vi "testpath2.vi"() -> (4 "Trajectory":T1[](array[typedef])=[{"t"=0.0, "velocity"=0.0, "acceleration"=2.3435826973687655, "pose"={"Translation2d"={"x"=0.0774192, "y"=0.185928}, "Rotation2d"={"Theta"=0.0}}, "curvature"=0.0}, {"t"=0.047106173277091413, "velocity"=0.11039721263144635, "acceleration"=-3.263996154199559, "pose"={"Translation2d"={"x"=0.08001852308776901, "y"=0.18586066416240327}, "Rotation2d"={"Theta"=-0.07810185233815048}}, "curvature"=-61.60474858569354}, {"t"=0.053259671361296806, "velocity"=0.0903122185497256, "acceleration"=-2.363925957623396, "pose"={"Translation2d"={"x"=0.08063303765779138, "y"=0.18579968634924657}, "Rotation2d"={"Theta"=-0.12154551781557862}}, "curvature"=-79.45370864068988}, {"t"=0.06060253182111065, "velocity"=0.07295424010556517, "acceleration"=-1.4416949338866047, "pose"={"Translation2d"={"x"=0.08122597127297766, "y"=0.1857117331972243}, "Rotation2d"={"Theta"=-0.1749375579100152}}, "curvature"=-99.06661763312775}, {"t"=0.0693110261969842, "velocity"=0.06039924788208828, "acceleration"=-0.9104988700910287, "pose"={"Translation2d"={"x"=0.08179438323477223, "y"=0.18559312894960375}, "Rotation2d"={"Theta"=-0.23853145947540738}}, "curvature"=-120.27826003101855}, {"t"=0.07938804352490185, "velocity"=0.05122413499113154, "acceleration"=-0.5792120596634627, "pose"={"Translation2d"={"x"=0.08233575624007373, "y"=0.18544072707720197}, "Rotation2d"={"Theta"=-0.31235747491337}}, "curvature"=-142.35551992491696}, {"t"=0.09077921007888227, "velocity"=0.04462623394943099, "acceleration"=-0.4038192359290258, "pose"={"Translation2d"={"x"=0.08284798009679452, "y"=0.18525188992348018}, "Rotation2d"={"Theta"=-0.3960059769552128}}, "curvature"=-163.8427702789242}, {"t"=0.09695072372373545, "velocity"=0.042134058024840826, "acceleration"=-0.31270644647916435, "pose"={"Translation2d"={"x"=0.08309260897132852, "y"=0.1851431179841045}, "Rotation2d"={"Theta"=-0.44121092624603003}}, "curvature"=-173.70999654118847}, {"t"=0.1033891694247334, "velocity"=0.0401207145488327, "acceleration"=-0.23490831082187247, "pose"={"Translation2d"={"x"=0.08332933543942006, "y"=0.18502446834963807}, "Rotation2d"={"Theta"=-0.488410728551556}}, "curvature"=-182.57657050349928}, {"t"=0.11005992609071186, "velocity"=0.03855369836852396, "acceleration"=-0.16695995975553915, "pose"={"Translation2d"={"x"=0.08355800297536588, "y"=0.18489574536915074}, "Rotation2d"={"Theta"=-0.5373459655625522}}, "curvature"=-190.11843445708558}, {"t"=0.116921657984853, "velocity"=0.037408063887624854, "acceleration"=-0.10600567598132761, "pose"={"Translation2d"={"x"=0.08377847744456844, "y"=0.18475678137970777}, "Rotation2d"={"Theta"=-0.5877071696426507}}, "curvature"=-196.03207220702802}, {"t"=0.12392714615426638, "velocity"=0.036665442378646995, "acceleration"=-0.0496073097812525, "pose"={"Translation2d"={"x"=0.0839906465946472, "y"=0.18460743607027907}, "Rotation2d"={"Theta"=-0.6391410543429555}}, "curvature"=-200.06281680826004}, {"t"=0.1310246385654173, "velocity"=0.03631335487393694, "acceleration"=0.004395319498262556, "pose"={"Translation2d"={"x"=0.08419441954654981, "y"=0.18444759584564838}, "Rotation2d"={"Theta"=-0.6912605824921103}}, "curvature"=-202.03146098771143}, {"t"=0.13815963801809006, "velocity"=0.03634471547615137, "acceleration"=0.05799027336927698, "pose"={"Translation2d"={"x"=0.08438972628566341, "y"=0.18427717319032236}, "Rotation2d"={"Theta"=-0.7436582689510874}}, "curvature"=-201.85456553695633}, {"t"=0.14527697526679556, "velocity"=0.03675745180886514, "acceleration"=0.11307728618805102, "pose"={"Translation2d"={"x"=0.0845765171529258, "y"=0.18409610603243998}, "Rotation2d"={"Theta"=-0.7959215893197124}}, "curvature"=-199.55457553174037}, {"t"=0.1523229647059073, "velocity"=0.037554193173149564, "acceleration"=0.17153717059604345, "pose"={"Translation2d"={"x"=0.08475476233593672, "y"=0.18390435710768158}, "Rotation2d"={"Theta"=-0.8476489989740198}}, "curvature"=-195.25769330622686}, {"t"=0.15924742526920344, "velocity"=0.038741995546081265, "acceleration"=0.23529206064245542, "pose"={"Translation2d"={"x"=0.08492445136006903, "y"=0.18370191332317803}, "Rotation2d"={"Theta"=-0.8984649589344123}}, "curvature"=-189.17993139104587}, {"t"=0.1660053740784075, "velocity"=0.04033208724711512, "acceleration"=0.3063602871556492, "pose"={"Translation2d"={"x"=0.08508559257958, "y"=0.1834887851214201}, "Rotation2d"={"Theta"=-0.9480325468739267}}, "curvature"=-181.6041156418403}, {"t"=0.17255825778502296, "velocity"=0.042339630581171406, "acceleration"=0.386908937568493, "pose"={"Translation2d"={"x"=0.0852382126687225, "y"=0.1832650058441675}, "Rotation2d"={"Theta"=-0.9960626519615907}}, "curvature"=-172.8521201807349}, {"t"=0.1788746609843625, "velocity"=0.0447835034322821, "acceleration"=0.47930689894890155, "pose"={"Translation2d"={"x"=0.08538235611285627, "y"=0.1830306310963581}, "Rotation2d"={"Theta"=-1.042319298697744}}, "curvature"=-163.2569342559984}, {"t"=0.18493050448955045, "velocity"=0.04768611100327358, "acceleration"=0.6490919973330421, "pose"={"Translation2d"={"x"=0.0855180846995591, "y"=0.18278573811001714}, "Rotation2d"={"Theta"=-1.0866211858450743}}, "curvature"=-153.1383845294613}, {"t"=0.19615830692266117, "velocity"=0.0549739877102422, "acceleration"=0.941459206443059, "pose"={"Translation2d"={"x"=0.08576462790874101, "y"=0.18226481066873368}, "Rotation2d"={"Theta"=-1.168895958568751}}, "curvature"=-132.44212851381863}, {"t"=0.20622279984151345, "velocity"=0.06444929722687665, "acceleration"=1.3418311536022953, "pose"={"Translation2d"={"x"=0.0859786633034792, "y"=0.18170324974681615}, "Rotation2d"={"Theta"=-1.2424085833564584}}, "curvature"=-112.53274117550998}, {"t"=0.21513918561432827, "velocity"=0.07641358143437582, "acceleration"=1.8923758205411287, "pose"={"Translation2d"={"x"=0.08616125615759282, "y"=0.18110238689435}, "Rotation2d"={"Theta"=-1.3072572259381148}}, "curvature"=-94.44693395075514}, {"t"=0.22297099217614624, "velocity"=0.09123430280311551, "acceleration"=2.6528140193058642, "pose"={"Translation2d"={"x"=0.08631369972706873, "y"=0.18046383863010146}, "Rotation2d"={"Theta"=-1.363907802949199}}, "curvature"=-78.62059191289242}, {"t"=0.22980662803577084, "velocity"=0.10936797344239757, "acceleration"=3.652890312976089, "pose"={"Translation2d"={"x"=0.0864374989656209, "y"=0.1797894860866117}, "Rotation2d"={"Theta"=-1.4130182829288853}}, "curvature"=-65.0912298694915}, {"t"=0.23575071787636012, "velocity"=0.1310810816405457, "acceleration"=4.389436457462054, "pose"={"Translation2d"={"x"=0.08653435424024987, "y"=0.17908145465529096}, "Rotation2d"={"Theta"=-1.4553132146872143}}, "curvature"=-53.67673857261736}, {"t"=0.24564788073800228, "velocity"=0.17452404913087727, "acceleration"=4.999999999999998, "pose"={"Translation2d"={"x"=0.08665491372552997, "y"=0.17757395585970945}, "Rotation2d"={"Theta"=-1.5222489468742197}}, "curvature"=-36.06210546716506}, {"t"=0.2611381435219113, "velocity"=0.25197536305042223, "acceleration"=5.000000000000002, "pose"={"Translation2d"={"x"=0.0866654015927572, "y"=0.17427067852316036}, "Rotation2d"={"Theta"=-1.601097292473268}}, "curvature"=-14.158339729780822}, {"t"=0.27358680122956974, "velocity"=0.3142186515887145, "acceleration"=-4.755099044000396, "pose"={"Translation2d"={"x"=0.0865021887608069, "y"=0.17075028219178084}, "Rotation2d"={"Theta"=-1.6249193382438698}}, "curvature"=-2.6727087142999493e-14}, {"t"=0.28596110166702643, "velocity"=0.2553776274083906, "acceleration"=-5.000000000000002, "pose"={"Translation2d"={"x"=0.0863389759288566, "y"=0.16722988586040133}, "Rotation2d"={"Theta"=-1.6010972924732687}}, "curvature"=14.158339729780678}, {"t"=0.3011563859447309, "velocity"=0.17940120601986828, "acceleration"=-4.932206251410714, "pose"={"Translation2d"={"x"=0.08634946379608383, "y"=0.1639266085238522}, "Rotation2d"={"Theta"=-1.5222489468742206}}, "curvature"=36.062105467164734}, {"t"=0.31088799373988385, "velocity"=0.13140290921633757, "acceleration"=-3.711994416551717, "pose"={"Translation2d"={"x"=0.08647002328136393, "y"=0.16241910972827067}, "Rotation2d"={"Theta"=-1.4553132146872154}}, "curvature"=53.676738572616834}, {"t"=0.31682413838376733, "velocity"=0.10936797344239868, "acceleration"=-2.652814019305907, "pose"={"Translation2d"={"x"=0.08656687855599289, "y"=0.16171107829694997}, "Rotation2d"={"Theta"=-1.4130182829288873}}, "curvature"=65.09122986949086}, {"t"=0.3236597742433918, "velocity"=0.09123430280311662, "acceleration"=-1.8923758205411012, "pose"={"Translation2d"={"x"=0.08669067779454505, "y"=0.1610367257534602}, "Rotation2d"={"Theta"=-1.3639078029492022}}, "curvature"=78.62059191289143}, {"t"=0.33149158080521013, "velocity"=0.07641358143437649, "acceleration"=-1.3418311536023326, "pose"={"Translation2d"={"x"=0.08684312136402099, "y"=0.16039817748921165}, "Rotation2d"={"Theta"=-1.307257225938117}}, "curvature"=94.44693395075427}, {"t"=0.34040796657802436, "velocity"=0.06444929722687776, "acceleration"=-0.9414592064431023, "pose"={"Translation2d"={"x"=0.0870257142181346, "y"=0.1597973146367455}, "Rotation2d"={"Theta"=-1.2424085833564629}}, "curvature"=112.53274117550862}, {"t"=0.3504724594968764, "velocity"=0.05497398771024309, "acceleration"=-0.6490919973330328, "pose"={"Translation2d"={"x"=0.08723974961287277, "y"=0.15923575371482798}, "Rotation2d"={"Theta"=-1.1688959585687553}}, "curvature"=132.44212851381695}, {"t"=0.3617002619299876, "velocity"=0.047686111003274245, "acceleration"=-0.4793068989489879, "pose"={"Translation2d"={"x"=0.0874862928220547, "y"=0.1587148262735445}, "Rotation2d"={"Theta"=-1.0866211858450798}}, "curvature"=153.13838452945902}, {"t"=0.3677561054351754, "velocity"=0.04478350343228232, "acceleration"=-0.38690893756843653, "pose"={"Translation2d"={"x"=0.08762202140875751, "y"=0.15846993328720355}, "Rotation2d"={"Theta"=-1.0423192986977496}}, "curvature"=163.2569342559969}, {"t"=0.37407250863451474, "velocity"=0.04233963058117207, "acceleration"=-0.30636028715561286, "pose"={"Translation2d"={"x"=0.08776616485289127, "y"=0.15823555853939414}, "Rotation2d"={"Theta"=-0.9960626519616004}}, "curvature"=172.8521201807327}, {"t"=0.38062539234113096, "velocity"=0.04033208724711579, "acceleration"=-0.23529206064256067, "pose"={"Translation2d"={"x"=0.0879187849420338, "y"=0.1580117792621415}, "Rotation2d"={"Theta"=-0.9480325468739346}}, "curvature"=181.60411564183696}, {"t"=0.3873833411503339, "velocity"=0.03874199554608149, "acceleration"=-0.1715371705960183, "pose"={"Translation2d"={"x"=0.08807992616154474, "y"=0.1577986510603836}, "Rotation2d"={"Theta"=-0.8984649589344227}}, "curvature"=189.17993139104385}, {"t"=0.3943078017136297, "velocity"=0.03755419317315001, "acceleration"=-0.11307728618807471, "pose"={"Translation2d"={"x"=0.08824961518567706, "y"=0.15759620727588008}, "Rotation2d"={"Theta"=-0.8476489989740267}}, "curvature"=195.25769330622353}, {"t"=0.40135379115274195, "velocity"=0.03675745180886536, "acceleration"=-0.05799027336924636, "pose"={"Translation2d"={"x"=0.08842786036868798, "y"=0.15740445835112166}, "Rotation2d"={"Theta"=-0.795921589319721}}, "curvature"=199.55457553173815}, {"t"=0.4084711284014474, "velocity"=0.03634471547615181, "acceleration"=-0.004395319498231251, "pose"={"Translation2d"={"x"=0.08861465123595037, "y"=0.15722339119323928}, "Rotation2d"={"Theta"=-0.7436582689510949}}, "curvature"=201.8545655369545}, {"t"=0.41560612785412043, "velocity"=0.03631335487393761, "acceleration"=0.04960730978122319, "pose"={"Translation2d"={"x"=0.088809957975064, "y"=0.15705296853791326}, "Rotation2d"={"Theta"=-0.6912605824921199}}, "curvature"=202.03146098770893}, {"t"=0.4227036202652711, "velocity"=0.03666544237864744, "acceleration"=0.10600567598136021, "pose"={"Translation2d"={"x"=0.08901373092696659, "y"=0.15689312831328253}, "Rotation2d"={"Theta"=-0.6391410543429665}}, "curvature"=200.06281680825916}, {"t"=0.4297091084346844, "velocity"=0.03740806388762552, "acceleration"=0.16695995975550962, "pose"={"Translation2d"={"x"=0.08922590007704534, "y"=0.15674378300385383}, "Rotation2d"={"Theta"=-0.587707169642665}}, "curvature"=196.0320722070255}, {"t"=0.4365708403288254, "velocity"=0.0385536983685244, "acceleration"=0.23490831082185235, "pose"={"Translation2d"={"x"=0.0894463745462479, "y"=0.15660481901441087}, "Rotation2d"={"Theta"=-0.5373459655625644}}, "curvature"=190.1184344570844}, {"t"=0.44324159699480353, "velocity"=0.040120714548832925, "acceleration"=0.31270644647914475, "pose"={"Translation2d"={"x"=0.0896750420821937, "y"=0.15647609603392354}, "Rotation2d"={"Theta"=-0.48841072855157025}}, "curvature"=182.57657050349698}, {"t"=0.4496800426958012, "velocity"=0.042134058024840826, "acceleration"=0.4038192359289669, "pose"={"Translation2d"={"x"=0.08991176855028524, "y"=0.15635744639945712}, "Rotation2d"={"Theta"=-0.4412109262460405}}, "curvature"=173.70999654118788}, {"t"=0.4558515563406553, "velocity"=0.04462623394943099, "acceleration"=0.5792120596635256, "pose"={"Translation2d"={"x"=0.09015639742481926, "y"=0.1562486744600814}, "Rotation2d"={"Theta"=-0.39600597695523054}}, "curvature"=163.8427702789235}, {"t"=0.4672427228946352, "velocity"=0.05122413499113199, "acceleration"=0.9104988700909966, "pose"={"Translation2d"={"x"=0.09066862128154003, "y"=0.15605983730635964}, "Rotation2d"={"Theta"=-0.31235747491338145}}, "curvature"=142.35551992491614}, {"t"=0.47731974022255297, "velocity"=0.0603992478820885, "acceleration"=1.4416949338865988, "pose"={"Translation2d"={"x"=0.09120999428684154, "y"=0.15590743543395782}, "Rotation2d"={"Theta"=-0.23853145947542465}}, "curvature"=120.27826003101823}, {"t"=0.4860282345984264, "velocity"=0.07295424010556517, "acceleration"=2.3639259576235054, "pose"={"Translation2d"={"x"=0.09177840624863609, "y"=0.15578883118633724}, "Rotation2d"={"Theta"=-0.17493755791003093}}, "curvature"=99.06661763312779}, {"t"=0.4933710950582401, "velocity"=0.09031221854972604, "acceleration"=3.0164280995608284, "pose"={"Translation2d"={"x"=0.09237133986382236, "y"=0.15570087803431498}, "Rotation2d"={"Theta"=-0.1215455178155994}}, "curvature"=79.45370864068965}, {"t"=0.4995676187072388, "velocity"=0.10900358660415899, "acceleration"=3.2099466552372213, "pose"={"Translation2d"={"x"=0.09298585443384472, "y"=0.15563990022115828}, "Rotation2d"={"Theta"=-0.07810185233816763}}, "curvature"=61.60474858569303}, {"t"=0.5182710790606299, "velocity"=0.16904069660688842, "acceleration"=-3.716363985732206, "pose"={"Translation2d"={"x"=0.09558517752161375, "y"=0.1555725643835615}, "Rotation2d"={"Theta"=-1.8307092179778333e-14}}, "curvature"=-1.7250053967029693e-12}, {"t"=0.5377224922029448, "velocity"=0.09675216533319107, "acceleration"=-2.770464533483307, "pose"={"Translation2d"={"x"=0.09816917506467329, "y"=0.1556453832888355}, "Rotation2d"={"Theta"=0.08595677451778284}}, "curvature"=70.17784975737536}, {"t"=0.5446559894788898, "velocity"=0.07754315703718229, "acceleration"=-2.0078311841616534, "pose"={"Translation2d"={"x"=0.09876980402437249, "y"=0.1557113264441974}, "Rotation2d"={"Theta"=0.1350468581629947}}, "curvature"=93.02774184231959}, {"t"=0.5530595181598164, "velocity"=0.060670290094621215, "acceleration"=-1.1912172586961445, "pose"={"Translation2d"={"x"=0.09934270232277766, "y"=0.15580644150438278}, "Rotation2d"={"Theta"=0.19658385081852184}}, "curvature"=119.72761813837175}, {"t"=0.5632492336568042, "velocity"=0.04853212513340566, "acceleration"=-0.8124403499649132, "pose"={"Translation2d"={"x"=0.09988408692354683, "y"=0.15593470353810518}, "Rotation2d"={"Theta"=0.2715148453026896}}, "curvature"=150.41695984182707}, {"t"=0.5690825133830074, "velocity"=0.04379293331120593, "acceleration"=-0.6349231723740711, "pose"={"Translation2d"={"x"=0.10014192836966991, "y"=0.15601234978286024}, "Rotation2d"={"Theta"=0.3142341701670356}}, "curvature"=167.0170658151397}, {"t"=0.5753905930993192, "velocity"=0.03978778732613675, "acceleration"=-0.4948018649167662, "pose"={"Translation2d"={"x"=0.10039071755097403, "y"=0.15609951529223298}, "Rotation2d"={"Theta"=0.36050711576775285}}, "curvature"=184.12921053172292}, {"t"=0.5821688812682085, "velocity"=0.03643387769922701, "acceleration"=-0.38270215664740254, "pose"={"Translation2d"={"x"=0.10063013081876065, "y"=0.15619653959569954}, "Rotation2d"={"Theta"=0.4102979234949966}}, "curvature"=201.35329274080783}, {"t"=0.5894020159674006, "velocity"=0.03366574145052503, "acceleration"=-0.29170994164656977, "pose"={"Translation2d"={"x"=0.10085987584071117, "y"=0.156303729204168}, "Rotation2d"={"Theta"=0.46349009309414674}}, "curvature"=218.15424122373147}, {"t"=0.5970616394795439, "velocity"=0.03143135312276302, "acceleration"=-0.2165495287954919, "pose"={"Translation2d"={"x"=0.101079690949347, "y"=0.1564213582978653}, "Rotation2d"={"Theta"=0.5198699448216428}}, "curvature"=233.87405185452747}, {"t"=0.6051047522811616, "velocity"=0.029689620835523733, "acceleration"=-0.1530548516883707, "pose"={"Translation2d"={"x"=0.10128934449048972, "y"=0.15654966941422405}, "Rotation2d"={"Theta"=0.5791145438826865}}, "curvature"=247.7688931629093}, {"t"=0.6134730769029672, "velocity"=0.028408808151653142, "acceleration"=-0.09781653921956363, "pose"={"Translation2d"={"x"=0.101488634171721, "y"=0.15668887413576937}, "Rotation2d"={"Theta"=0.6407871610915417}}, "curvature"=259.0738230220722}, {"t"=0.6220938211947187, "velocity"=0.027565556779537204, "acceleration"=-0.047936377452372066, "pose"={"Translation2d"={"x"=0.10167738641084273, "y"=0.15683915377800575}, "Rotation2d"={"Theta"=0.7043431189362696}}, "curvature"=267.090182633088}, {"t"=0.630882063228603, "velocity"=0.027144280292258127, "acceleration"=-0.0008482709654389815, "pose"={"Translation2d"={"x"=0.10185545568433707, "y"=0.1570006600773038}, "Rotation2d"={"Theta"=0.7691476236098189}}, "curvature"=271.2816109003646}, {"t"=0.6397446945257157, "velocity"=0.027136762379451396, "acceleration"=0.04581900522136835, "pose"={"Translation2d"={"x"=0.1020227238758265, "y"=0.1571735158787871}, "Rotation2d"={"Theta"=0.8345050811793381}}, "curvature"=271.35759117150434}, {"t"=0.6485855194035324, "velocity"=0.02754184018068928, "acceleration"=0.094352224676927, "pose"={"Translation2d"={"x"=0.10217909962453388, "y"=0.1573578158242192}, "Rotation2d"={"Theta"=0.8996969187800623}}, "curvature"=267.3227413392821}, {"t"=0.6573108246167323, "velocity"=0.028365092138539882, "acceleration"=0.1470463333023926, "pose"={"Translation2d"={"x"=0.10232451767374248, "y"=0.15755362703989023}, "Rotation2d"={"Theta"=0.9640228667260538}}, "curvature"=259.4776945641172}, {"t"=0.665834611580665, "velocity"=0.02961848375743692, "acceleration"=0.20628477568028816, "pose"={"Translation2d"={"x"=0.10245893821925611, "y"=0.15776098982450382}, "Rotation2d"={"Theta"=1.0268397706121175}}, "curvature"=248.3711315953599}, {"t"=0.6740827724095978, "velocity"=0.03131995376380825, "acceleration"=0.27461105367069044, "pose"={"Translation2d"={"x"=0.10258234625785909, "y"=0.15797991833706393}, "Rotation2d"={"Theta"=1.0875926461201102}}, "curvature"=234.7164907677842}, {"t"=0.6819957548250865, "velocity"=0.033492946202603235, "acceleration"=0.35479413019379735, "pose"={"Translation2d"={"x"=0.10269475093577635, "y"=0.15821040128476174}, "Rotation2d"={"Theta"=1.1458346067318121}}, "curvature"=219.2950955053735}, {"t"=0.6895295990710837, "velocity"=0.03616590991887736, "acceleration"=0.44989007893007565, "pose"={"Translation2d"={"x"=0.1027961848971335, "y"=0.1584524026108624}, "Rotation2d"={"Theta"=1.201234763455286}}, "curvature"=202.86726425582916}, {"t"=0.6966555302806612, "velocity"=0.03937179567320448, "acceleration"=0.5633026373286869, "pose"={"Translation2d"={"x"=0.10288670363241685, "y"=0.15870586218259194}, "Rotation2d"={"Theta"=1.2535754049780008}}, "curvature"=186.10613248202148}, {"t"=0.7033584784246697, "velocity"=0.04314758404060193, "acceleration"=0.69884590081536, "pose"={"Translation2d"={"x"=0.1029663848269335, "y"=0.15897069647902398}, "Rotation2d"={"Theta"=1.3027411728436478}}, "curvature"=169.55964344713635}, {"t"=0.7096349582300072, "velocity"=0.047533876224112426, "acceleration"=0.8608132364314004, "pose"={"Translation2d"={"x"=0.1030353277092714, "y"=0.1592467992789667}, "Rotation2d"={"Theta"=1.3487034150678574}}, "curvature"=153.63837147221966}, {"t"=0.7154907009894446, "velocity"=0.05257457710057345, "acceleration"=1.1710273135760545, "pose"={"Translation2d"={"x"=0.10309365239975934, "y"=0.15953404234884963}, "Rotation2d"={"Theta"=1.3915026250306544}}, "curvature"=138.62245564664414}, {"t"=0.7259394069127965, "velocity"=0.06481029712834241, "acceleration"=1.7215619926356163, "pose"={"Translation2d"={"x"=0.10317902823596548, "y"=0.16014133042958176}, "Rotation2d"={"Theta"=1.4680178073712176}}, "curvature"=111.88933562608142}, {"t"=0.7349184761898326, "velocity"=0.08026832152493002, "acceleration"=2.491621101203314, "pose"={"Translation2d"={"x"=0.10322386637448248, "y"=0.1607911207447828}, "Rotation2d"={"Theta"=1.5333858309580801}}, "curvature"=89.768286926723}, {"t"=0.7426047973908486, "velocity"=0.0994197216200079, "acceleration"=3.320618702108264, "pose"={"Translation2d"={"x"=0.10322981342353883, "y"=0.16148166514471396}, "Rotation2d"={"Theta"=1.5889293086419294}}, "curvature"=71.90243531656316}, {"t"=0.755075794176805, "velocity"=0.14083114678138683, "acceleration"=5.00000000000001, "pose"={"Translation2d"={"x"=0.10313295843700387, "y"=0.1629766148075767}, "Rotation2d"={"Theta"=1.675700032982173}}, "curvature"=46.28096736583443}, {"t"=0.7650105898872683, "velocity"=0.19050512533370356, "acceleration"=4.999999999999997, "pose"={"Translation2d"={"x"=0.1029066952555758, "y"=0.16460686722462275}, "Rotation2d"={"Theta"=1.7372462719476571}}, "curvature"=29.907284772497857}, {"t"=0.78087148876621, "velocity"=0.2698096197284119, "acceleration"=5.0, "pose"={"Translation2d"={"x"=0.1021549388228159, "y"=0.16817912604026272}, "Rotation2d"={"Theta"=1.808119721975475}}, "curvature"=11.392762400320894}, {"t"=0.7938746162185758, "velocity"=0.3348252569902407, "acceleration"=-4.87580343734334, "pose"={"Translation2d"={"x"=0.10117532587401734, "y"=0.17198618356164386}, "Rotation2d"={"Theta"=1.8300183745307927}}, "curvature"=0.33963534680191004}, {"t"=0.8224893227987234, "velocity"=0.1953055722881857, "acceleration"=-5.000000000000001, "pose"={"Translation2d"={"x"=0.0994219257031623, "y"=0.17936549989866496}, "Rotation2d"={"Theta"=1.7435098835081544}}, "curvature"=-28.695429879989835}, {"t"=0.8321101400212955, "velocity"=0.1472014861753257, "acceleration"=-3.737334957184971, "pose"={"Translation2d"={"x"=0.09918347402379073, "y"=0.18099575231571102}, "Rotation2d"={"Theta"=1.6841931776688102}}, "curvature"=-44.681687822810645}, {"t"=0.8441274989785668, "velocity"=0.10228859045127559, "acceleration"=-2.6661130356198317, "pose"={"Translation2d"={"x"=0.09907192127589325, "y"=0.18249070197857378}, "Rotation2d"={"Theta"=1.6001259710533695}}, "curvature"=-69.80228261669235}, {"t"=0.851607676765601, "velocity"=0.08234559094450966, "acceleration"=-1.838290850505451, "pose"={"Translation2d"={"x"=0.09906961498842175, "y"=0.1831812463785049}, "Rotation2d"={"Theta"=1.5461204056689324}}, "curvature"=-87.42865136904975}, {"t"=0.8603672639780126, "velocity"=0.06624292191772896, "acceleration"=-1.2483239554812005, "pose"={"Translation2d"={"x"=0.09910561901369269, "y"=0.18383103669370598}, "Rotation2d"={"Theta"=1.4823867426308317}}, "curvature"=-109.4051223052071}, {"t"=0.8705912402278141, "velocity"=0.053480087444830904, "acceleration"=-0.8318978310404131, "pose"={"Translation2d"={"x"=0.09918159830382774, "y"=0.1844383247744381}, "Rotation2d"={"Theta"=1.4075396162448133}}, "curvature"=-136.224917991435}, {"t"=0.8824436182677277, "velocity"=0.04362011986075576, "acceleration"=-0.5998518589850211, "pose"={"Translation2d"={"x"=0.09929892660045758, "y"=0.1850016706442638}, "Rotation2d"={"Theta"=1.32036282084814}}, "curvature"=-167.69054870808148}, {"t"=0.8890509169113168, "velocity"=0.0396567194865296, "acceleration"=-0.47956032045977043, "pose"={"Translation2d"={"x"=0.09937344116172195, "y"=0.18526650494069583}, "Rotation2d"={"Theta"=1.2719031149668187}}, "curvature"=-184.74761053814296}, {"t"=0.8960938025586663, "velocity"=0.036279230988525146, "acceleration"=-0.37909202474885084, "pose"={"Translation2d"={"x"=0.09945866558544372, "y"=0.18551996451242536}, "Rotation2d"={"Theta"=1.2201732587521341}}, "curvature"=-202.22429069675667}, {"t"=0.9035615184878253, "velocity"=0.03344827943669104, "acceleration"=-0.29482779660640884, "pose"={"Translation2d"={"x"=0.09955468040193201, "y"=0.185761965838526}, "Rotation2d"={"Theta"=1.165256443743712}}, "curvature"=-219.59191832860543}, {"t"=0.9114297200747205, "velocity"=0.03112851489957169, "acceleration"=-0.22353499147615324, "pose"={"Translation2d"={"x"=0.09966154403160041, "y"=0.18599244878622384}, "Rotation2d"={"Theta"=1.107337414513009}}, "curvature"=-236.1782993686969}, {"t"=0.9196586026064402, "velocity"=0.02928907171298545, "acceleration"=-0.16230327944072007, "pose"={"Translation2d"={"x"=0.09977929213342746, "y"=0.18621137729878398}, "Rotation2d"={"Theta"=1.0467162157481573}}, "curvature"=-251.19803495847782}, {"t"=0.9281920121728392, "velocity"=0.027904071355548066, "acceleration"=-0.10848051716776347, "pose"={"Translation2d"={"x"=0.09990793695341624, "y"=0.18641874008339754}, "Rotation2d"={"Theta"=0.9838145805699998}}, "curvature"=-263.81388801484485}, {"t"=0.936957981706207, "velocity"=0.026953134447091465, "acceleration"=-0.05960573119375002, "pose"={"Translation2d"={"x"=0.10004746667305481, "y"=0.18661455129906857}, "Rotation2d"={"Theta"=0.9191717247022588}}, "curvature"=-273.22659999761464}, {"t"=0.9458709774559114, "velocity"=0.02642186881830355, "acceleration"=-0.01333662403488536, "pose"={"Translation2d"={"x"=0.10019784475777607, "y"=0.18679885124450066}, "Rotation2d"={"Theta"=0.8534274890519126}}, "curvature"=-278.7802541019173}, {"t"=0.9548358472267702, "velocity"=0.0263023077206479, "acceleration"=0.032631042753267656, "pose"={"Translation2d"={"x"=0.10035900930541793, "y"=0.186971707045984}, "Rotation2d"={"Theta"=0.7872929428384702}}, "curvature"=-280.06102787176684}, {"t"=0.9637530921406602, "velocity"=0.026593286720674403, "acceleration"=0.08065556213396426, "pose"={"Translation2d"={"x"=0.10053087239468307, "y"=0.18713321334528205}, "Rotation2d"={"Theta"=0.7215112626164386}}, "curvature"=-276.9640671721246}, {"t"=0.9725247548891591, "velocity"=0.027300770110504136, "acceleration"=0.13325800247006186, "pose"={"Translation2d"={"x"=0.10071331943359957, "y"=0.18728349298751842}, "Rotation2d"={"Theta"=0.6568140938882268}}, "curvature"=-269.7095376623658}, {"t"=0.9810600533034425, "velocity"=0.028438166927677422, "acceleration"=0.19325589530700452, "pose"={"Translation2d"={"x"=0.10090620850798024, "y"=0.18742269770906375}, "Rotation2d"={"Theta"=0.5938797909916752}}, "curvature"=-258.8032881521894}, {"t"=0.98927995564165, "velocity"=0.030026711513383875, "acceleration"=0.26393579962518937, "pose"={"Translation2d"={"x"=0.10110936972988338, "y"=0.18755100882542255}, "Rotation2d"={"Theta"=0.5332994383480658}}, "curvature"=-244.95392013920517}, {"t"=0.9971201652520616, "velocity"=0.03209602350613694, "acceleration"=0.3492878526136228, "pose"={"Translation2d"={"x"=0.1013226045860724, "y"=0.18766863791911984}, "Rotation2d"={"Theta"=0.4755545834395076}}, "curvature"=-228.9691317443559}, {"t"=1.0045323503304004, "velocity"=0.03468500971532462, "acceleration"=0.4543407293916066, "pose"={"Translation2d"={"x"=0.10154568528647583, "y"=0.18777582752758828}, "Rotation2d"={"Theta"=0.42100792629471184}}, "curvature"=-211.65596129145138}, {"t"=1.0114837920876667, "velocity"=0.03784333283364427, "acceleration"=0.5856615279390037, "pose"={"Translation2d"={"x"=0.10177835411264778, "y"=0.18787285183105482}, "Rotation2d"={"Theta"=0.36990573115040026}}, "curvature"=-193.74308696394925}, {"t"=1.017955843288908, "velocity"=0.04163376422906273, "acceleration"=0.7521310839980412, "pose"={"Translation2d"={"x"=0.10202032276622766, "y"=0.18796001734042758}, "Rotation2d"={"Theta"=0.32238910169977497}}, "curvature"=-175.8331728878996}, {"t"=1.0239416646425101, "velocity"=0.04613588653236622, "acceleration"=1.1077846736780808, "pose"={"Translation2d"={"x"=0.10227127171740036, "y"=0.18803766358518265}, "Rotation2d"={"Theta"=0.27851067991036266}}, "curvature"=-158.3840879145007}, {"t"=1.0343945509271988, "velocity"=0.05771543375424404, "acceleration"=1.875703575631341, "pose"={"Translation2d"={"x"=0.10279867232675113, "y"=0.18816592561890508}, "Rotation2d"={"Theta"=0.2015502334025794}}, "curvature"=-126.00976743551827}, {"t"=1.0430080981166385, "velocity"=0.0738718950163455, "acceleration"=2.467321293545936, "pose"={"Translation2d"={"x"=0.1033573503145702, "y"=0.18826104067909044}, "Rotation2d"={"Theta"=0.13838031277314014}}, "curvature"=-97.79899632033535}, {"t"=1.0501433849548638, "velocity"=0.09147694016785679, "acceleration"=3.253927227246253, "pose"={"Translation2d"={"x"=0.1039435586528987, "y"=0.18832698383445234}, "Rotation2d"={"Theta"=0.08802956458905108}}, "curvature"=-73.67639668026254}, {"t"=1.061422853396756, "velocity"=0.12817950963979463, "acceleration"=4.289933588494223, "pose"={"Translation2d"={"x"=0.10518074616443314, "y"=0.1883902483890585}, "Rotation2d"={"Theta"=0.02220021162876268}}, "curvature"=-34.51484544057754}, {"t"=1.0701857218783168, "velocity"=0.16577163347039933, "acceleration"=-3.6515252670326634, "pose"={"Translation2d"={"x"=0.10646863832853012, "y"=0.18839980273972629}, "Rotation2d"={"Theta"=2.9426732770626766e-14}}, "curvature"=2.836228175771673e-12}, {"t"=1.0895659679151655, "velocity"=0.09500417538553715, "acceleration"=-2.7207734633231833, "pose"={"Translation2d"={"x"=0.10899459853675333, "y"=0.1883290945273587}, "Rotation2d"={"Theta"=-0.0854011037217413}}, "curvature"=-71.36631849517777}, {"t"=1.096462169489461, "velocity"=0.07624117314446655, "acceleration"=-1.9934423590169708, "pose"={"Translation2d"={"x"=0.10958158763091988, "y"=0.1882650627678044}, "Rotation2d"={"Theta"=-0.13420095994761355}}, "curvature"=-94.66724584083127}, {"t"=1.1048161257058737, "velocity"=0.05958804295729614, "acceleration"=-1.182546116555915, "pose"={"Translation2d"={"x"=0.11014137547317829, "y"=0.18817270466588526}, "Rotation2d"={"Theta"=-0.19540776415030497}}, "curvature"=-121.95621322978805}, {"t"=1.1149542882556525, "velocity"=0.04759919820504277, "acceleration"=-0.8065776143012836, "pose"={"Translation2d"={"x"=0.11067024973438806, "y"=0.18804816037227076}, "Rotation2d"={"Theta"=-0.26999442698449216}}, "curvature"=-153.42344179030619}, {"t"=1.120762814474175, "velocity"=0.04291417098510042, "acceleration"=-0.6304787092517313, "pose"={"Translation2d"={"x"=0.11092208018326222, "y"=0.1879727647433057}, "Rotation2d"={"Theta"=-0.31254883046411347}}, "curvature"=-170.49808634267168}, {"t"=1.1270480150924895, "velocity"=0.03895148581187735, "acceleration"=-0.49156069935597885, "pose"={"Translation2d"={"x"=0.11116503003703918, "y"=0.1878881257704365}, "Rotation2d"={"Theta"=-0.3586707903789192}}, "curvature"=-188.1464616868444}, {"t"=1.1338064055172965, "velocity"=0.03562932668813845, "acceleration"=-0.38052086652499706, "pose"={"Translation2d"={"x"=0.11139878151500279, "y"=0.18779391376562116}, "Rotation2d"={"Theta"=-0.4083328422356733}}, "curvature"=-205.96732356101813}, {"t"=1.1410238482082429, "velocity"=0.03288293914128504, "acceleration"=-0.2905024408316854, "pose"={"Translation2d"={"x"=0.11162304753029403, "y"=0.1876898311023257}, "Rotation2d"={"Theta"=-0.46142764864700314}}, "curvature"=-223.4184511929345}, {"t"=1.1486732571737868, "velocity"=0.030660767165874736, "acceleration"=-0.21627825514852766, "pose"={"Translation2d"={"x"=0.11183757105163113, "y"=0.18757561154757615}, "Rotation2d"={"Theta"=-0.5177510355035749}}, "curvature"=-239.82676442283454}, {"t"=1.1567128479476634, "velocity"=0.02892197850119249, "acceleration"=-0.15372576433392146, "pose"={"Translation2d"={"x"=0.11204212446502954, "y"=0.1874510195940104}, "Rotation2d"={"Theta"=-0.5769891409471083}}, "curvature"=-254.42417091056544}, {"t"=1.1650853706883255, "velocity"=0.027634906043481067, "acceleration"=-0.09947696645275515, "pose"={"Translation2d"={"x"=0.11223650893552208, "y"=0.18731584979193017}, "Rotation2d"={"Theta"=-0.6387129060337343}}, "curvature"=-266.41245216187883}, {"t"=1.173718733856308, "velocity"=0.02677608526524522, "acceleration"=-0.05067511975014293, "pose"={"Translation2d"={"x"=0.11242055376887898, "y"=0.1871699260813528}, "Rotation2d"={"Theta"=-0.7023828897284227}}, "curvature"=-275.05292254920397}, {"t"=1.18252826789836, "velocity"=0.026329661072721278, "acceleration"=-0.004797565338293713, "pose"={"Translation2d"={"x"=0.11259411577332792, "y"=0.1870131011240634}, "Rotation2d"={"Theta"=-0.7673662089061012}}, "curvature"=-279.7669845299291}, {"t"=1.191420595654658, "velocity"=0.026286999549300916, "acceleration"=0.04047994497850446, "pose"={"Translation2d"={"x"=0.11275707862127413, "y"=0.18684525563566656}, "Rotation2d"={"Theta"=-0.8329653207785566}}, "curvature"=-280.22585487406246}, {"t"=1.2002987300489298, "velocity"=0.02664638594109281, "acceleration"=0.08739231833729783, "pose"={"Translation2d"={"x"=0.11290935221102039, "y"=0.1866662977176383}, "Rotation2d"={"Theta"=-0.8984558337431857}}, "curvature"=-276.4062167927869}, {"t"=1.2090677192116492, "velocity"=0.027412728233497496, "acceleration"=0.13817658257504883, "pose"={"Translation2d"={"x"=0.11305087202848717, "y"=0.18647616218937801}, "Rotation2d"={"Theta"=-0.9631283452570846}}, "curvature"=-268.59583728225317}, {"t"=1.2176400167928687, "velocity"=0.02859721901808676, "acceleration"=0.19515119988682209, "pose"={"Translation2d"={"x"=0.11318159850893261, "y"=0.1862748099202605}, "Rotation2d"={"Theta"=-1.0263282697065548}}, "curvature"=-257.34731321790406}, {"t"=1.2259398283000917, "velocity"=0.030216937192555804, "acceleration"=0.2607867143590383, "pose"={"Translation2d"={"x"=0.11330151639867268, "y"=0.18606222716168763}, "Rotation2d"={"Theta"=-1.0874881475790634}}, "curvature"=-243.39310723257265}, {"t"=1.2339059430997878, "velocity"=0.032294394097375445, "acceleration"=0.33777028458058916, "pose"={"Translation2d"={"x"=0.11341063411680115, "y"=0.18583842487914046}, "Rotation2d"={"Theta"=-1.1461488074139536}}, "curvature"=-227.54438118828813}, {"t"=1.2414929062649822, "velocity"=0.034857044804785575, "acceleration"=0.4290664247446799, "pose"={"Translation2d"={"x"=0.11350898311690968, "y"=0.18560343808423113}, "Rotation2d"={"Theta"=-1.2019682666495493}}, "curvature"=-210.5966476375705}, {"t"=1.248670698187739, "velocity"=0.037936794322644074, "acceleration"=0.5379765174373194, "pose"={"Translation2d"={"x"=0.11359661724880796, "y"=0.18535732516675463}, "Rotation2d"={"Theta"=-1.2547195637493243}}, "curvature"=-193.2584432255869}, {"t"=1.2554232926419575, "velocity"=0.04156953157079113, "acceleration"=0.6682002217051316, "pose"={"Translation2d"={"x"=0.11367361212024363, "y"=0.1851001672267409}, "Rotation2d"={"Theta"=-1.3042802230553217}}, "curvature"=-176.10946914655926}, {"t"=1.2617465343181247, "velocity"=0.0457947230607012, "acceleration"=0.8239027139112283, "pose"={"Translation2d"={"x"=0.11374006445862243, "y"=0.18483206740650665}, "Rotation2d"={"Theta"=-1.3506165973360953}}, "curvature"=-159.58620878017567}, {"t"=1.2676457409083308, "velocity"=0.05065509538029511, "acceleration"=1.122391568580036, "pose"={"Translation2d"={"x"=0.1137960914727283, "y"=0.1845531502227073}, "Rotation2d"={"Theta"=-1.3937660908844118}}, "curvature"=-143.9881381698022}, {"t"=1.2781700699034757, "velocity"=0.06246751350940816, "acceleration"=1.6527080595663284, "pose"={"Translation2d"={"x"=0.11387743694046792, "y"=0.18396346469503988}, "Rotation2d"={"Theta"=-1.4709054934935915}}, "curvature"=-116.19731747125384}, {"t"=1.2872111565072826, "velocity"=0.07740979020675676, "acceleration"=2.395385233282257, "pose"={"Translation2d"={"x"=0.11391897156665912, "y"=0.1833325088817287}, "Rotation2d"={"Theta"=-1.5367982374777287}}, "curvature"=-93.19314674514915}, {"t"=1.29494734435199, "velocity"=0.09594094033186695, "acceleration"=3.204427407084343, "pose"={"Translation2d"={"x"=0.11392230524663283, "y"=0.1826619802615057}, "Rotation2d"={"Theta"=-1.5927777102801357}}, "curvature"=-74.61756469850788}, {"t"=1.3015976260182398, "velocity"=0.1172512851680278, "acceleration"=3.9635813891197857, "pose"={"Translation2d"={"x"=0.11388931430289642, "y"=0.18195385417950594}, "Rotation2d"={"Theta"=-1.640176953540165}}, "curvature"=-59.793915573356564}, {"t"=1.3073961780550554, "velocity"=0.14023431810499237, "acceleration"=4.888068532447168, "pose"={"Translation2d"={"x"=0.1138221210601756, "y"=0.18121036247292885}, "Rotation2d"={"Theta"=-1.6802112971716348}}, "curvature"=-47.99961164993872}, {"t"=1.3171441949421774, "velocity"=0.1878832927046974, "acceleration"=5.000000000000002, "pose"={"Translation2d"={"x"=0.11359472443802737, "y"=0.1796273637491305}, "Rotation2d"={"Theta"=-1.742227843591752}}, "curvature"=-31.015296379228783}, {"t"=1.332779334450521, "velocity"=0.26605899024641594, "acceleration"=4.999999999999998, "pose"={"Translation2d"={"x"=0.11284541269991404, "y"=0.17615864866727718}, "Rotation2d"={"Theta"=-1.8137452147475845}}, "curvature"=-11.860679682631737}, {"t"=1.3456030394623133, "velocity"=0.3301775153053772, "acceleration"=-4.910842396854063, "pose"={"Translation2d"={"x"=0.11187097444868144, "y"=0.17246194063926945}, "Rotation2d"={"Theta"=-1.8361458971072673}}, "curvature"=-0.4762604750853638}, {"t"=1.3738990866630907, "velocity"=0.19122008704841614, "acceleration"=-5.0, "pose"={"Translation2d"={"x"=0.11011795218492636, "y"=0.16529651752940838}, "Rotation2d"={"Theta"=-1.7507804064940407}}, "curvature"=29.308064752294065}, {"t"=1.383473390431305, "velocity"=0.14334856820734476, "acceleration"=-3.6369410802705238, "pose"={"Translation2d"={"x"=0.10987436072510647, "y"=0.16371351880561003}, "Rotation2d"={"Theta"=-1.691817044899504}}, "curvature"=45.74029558457744}, {"t"=1.3954555702468752, "velocity"=0.09977008620490979, "acceleration"=-2.6282295167646774, "pose"={"Translation2d"={"x"=0.10975464764669657, "y"=0.16226190101703314}, "Rotation2d"={"Theta"=-1.6080938154691242}}, "curvature"=71.63947680773273}, {"t"=1.4029083334522467, "velocity"=0.0801825139670942, "acceleration"=-1.8082331049564886, "pose"={"Translation2d"={"x"=0.10974701513166105, "y"=0.16159137239681015}, "Rotation2d"={"Theta"=-1.5542291838349456}}, "curvature"=89.86753946201071}, {"t"=1.4116472013487682, "velocity"=0.06438060373676247, "acceleration"=-1.2252120728170661, "pose"={"Translation2d"={"x"=0.10977681188574881, "y"=0.160960416583499}, "Rotation2d"={"Theta"=-1.4905873873528714}}, "curvature"=112.6559898532545}, {"t"=1.4218615793663387, "velocity"=0.05186582447331789, "acceleration"=-0.8981827251093194, "pose"={"Translation2d"={"x"=0.10984567217779234, "y"=0.16037073105583155}, "Rotation2d"={"Theta"=-1.4157492066313964}}, "curvature"=140.5574403023494}, {"t"=1.4276093804600978, "velocity"=0.046703248823539045, "acceleration"=-0.728181113418139, "pose"={"Translation2d"={"x"=0.10989518447559836, "y"=0.16009181387203217}, "Rotation2d"={"Theta"=-1.3737223202829194}}, "curvature"=156.42382455395153}, {"t"=1.4337884083995693, "velocity"=0.04220379737873281, "acceleration"=-0.5864376611457345, "pose"={"Translation2d"={"x"=0.10995494522993435, "y"=0.15982371405179796}, "Rotation2d"={"Theta"=-1.328453402042928}}, "curvature"=173.41803004450423}, {"t"=1.4404086718137454, "velocity"=0.03832142558595475, "acceleration"=-0.46836896326977173, "pose"={"Translation2d"={"x"=0.11002507520405308, "y"=0.15956655611178422}, "Rotation2d"={"Theta"=-1.279869924650177}}, "curvature"=191.2888242840875}, {"t"=1.4474714697875823, "velocity"=0.035013430221164876, "acceleration"=-0.3699268124373161, "pose"={"Translation2d"={"x"=0.1101056747926696, "y"=0.15932044319430771}, "Rotation2d"={"Theta"=-1.2279647766293003}}, "curvature"=209.6427298577038}, {"t"=1.454966780461978, "velocity"=0.03224071383515836, "acceleration"=-0.28752080273559205, "pose"={"Translation2d"={"x"=0.11019682338368111, "y"=0.15908545639939836}, "Rotation2d"={"Theta"=-1.1728156577163034}}, "curvature"=227.92819690681276}, {"t"=1.462870758005334, "velocity"=0.029968155867088564, "acceleration"=-0.217949762135638, "pose"={"Translation2d"={"x"=0.11029857871988713, "y"=0.15886165411685121}, "Rotation2d"={"Theta"=-1.1146035916342667}}, "curvature"=245.43836115499695}, {"t"=1.4711437402572525, "velocity"=0.02816506135313057, "acceleration"=-0.1583372842142787, "pose"={"Translation2d"={"x"=0.11041097626070939, "y"=0.15864907135827835}, "Rotation2d"={"Theta"=-1.0536275630080996}}, "curvature"=261.3416771795421}, {"t"=1.4797292513807108, "velocity"=0.026805654838250703, "acceleration"=-0.10606763240432845, "pose"={"Translation2d"={"x"=0.11053402854391213, "y"=0.15844771908916086}, "Rotation2d"={"Theta"=-0.990311702135687}}, "curvature"=274.7462241795335}, {"t"=1.4885544694757828, "velocity"=0.025869584849454563, "acceleration"=-0.05871901893181915, "pose"={"Translation2d"={"x"=0.11066772454732189, "y"=0.15825758356090058}, "Rotation2d"={"Theta"=-0.9252015770462404}}, "curvature"=284.79544429066965}, {"t"=1.4975324717729357, "velocity"=0.02534240536259813, "acceleration"=-0.01399167835129339, "pose"={"Translation2d"={"x"=0.11081202905054788, "y"=0.1580786256428723}, "Rotation2d"={"Theta"=-0.8589473364382797}}, "curvature"=290.7817808254249}, {"t"=1.5065662649819316, "velocity"=0.025216007433725762, "acceleration"=0.030371862176745982, "pose"={"Translation2d"={"x"=0.11096688199670174, "y"=0.1579107801544754}, "Rotation2d"={"Theta"=-0.7922736994181389}}, "curvature"=292.25428223149527}, {"t"=1.5155542182607735, "velocity"=0.02548898831196178, "acceleration"=0.07667758801603829, "pose"={"Translation2d"={"x"=0.11113219785411782, "y"=0.15775395519718605}, "Rotation2d"={"Theta"=-0.7259396414706821}}, "curvature"=289.09241796645773}, {"t"=1.5243961642741963, "velocity"=0.026166967405639063, "acceleration"=0.1273868144897145, "pose"={"Translation2d"={"x"=0.11130786497807316, "y"=0.15760803148660865}, "Rotation2d"={"Theta"=-0.6606931857136354}}, "curvature"=281.5249563277378}, {"t"=1.5329992537371506, "velocity"=0.02726288756709483, "acceleration"=0.18524710088810553, "pose"={"Translation2d"={"x"=0.11149374497250758, "y"=0.15747286168452843}, "Rotation2d"={"Theta"=-0.5972280125257533}}, "curvature"=270.0884443727916}, {"t"=1.5412827151394868, "velocity"=0.028797374777196127, "acceleration"=0.2534607445216884, "pose"={"Translation2d"={"x"=0.11168967205174363, "y"=0.1573482697309627}, "Rotation2d"={"Theta"=-0.5361481172995145}}, "curvature"=255.5379268738299}, {"t"=1.5491809561465237, "velocity"=0.030799268823251458, "acceleration"=0.3359133007071068, "pose"={"Translation2d"={"x"=0.11189545240220684, "y"=0.1572340501762131}, "Rotation2d"={"Theta"=-0.47794467568295046}}, "curvature"=238.73489308826373}, {"t"=1.5566448326241376, "velocity"=0.03330648420691684, "acceleration"=0.43749949252794257, "pose"={"Translation2d"={"x"=0.11211086354414561, "y"=0.1571299675129177}, "Rotation2d"={"Theta"=-0.42298643498378197}}, "curvature"=220.5394614081102}, {"t"=1.5636412686975967, "velocity"=0.03636742143855942, "acceleration"=0.5646092915946906, "pose"={"Translation2d"={"x"=0.11233565369335143, "y"=0.1570357555081023}, "Rotation2d"={"Theta"=-0.37152232606289437}}, "curvature"=201.72667864010563}, {"t"=1.5701516417247912, "velocity"=0.04004323854146086, "acceleration"=0.7258817451502695, "pose"={"Translation2d"={"x"=0.11256954112287879, "y"=0.15695111653523314}, "Rotation2d"={"Theta"=-0.3236932778807512}}, "curvature"=182.9355827769611}, {"t"=1.5761694240335946, "velocity"=0.044411436865709586, "acceleration"=1.0708055347703593, "pose"={"Translation2d"={"x"=0.11281221352476536, "y"=0.15687572090626808}, "Rotation2d"={"Theta"=-0.27954961563049985}}, "curvature"=164.64960250470264}, {"t"=1.5866680596250309, "velocity"=0.05565343396455669, "acceleration"=1.8162891580088538, "pose"={"Translation2d"={"x"=0.11332250727900264, "y"=0.15675117661265356}, "Rotation2d"={"Theta"=-0.2021844233802083}}, "curvature"=130.78885077236274}, {"t"=1.5953092300826401, "velocity"=0.07134829817921884, "acceleration"=2.3830331591858815, "pose"={"Translation2d"={"x"=0.1138634006173894, "y"=0.15665881851073443}, "Rotation2d"={"Theta"=-0.13874583430957563}}, "curvature"=101.36348330583021}, {"t"=1.6024634578187813, "velocity"=0.08839706010281079, "acceleration"=1.946002936893058, "pose"={"Translation2d"={"x"=0.11443122905506596, "y"=0.1565947867511801}, "Rotation2d"={"Theta"=-0.08822539249242686}}, "curvature"=76.26938445996804}, {"t"=1.6144610116874072, "velocity"=0.1117443351666894, "acceleration"=-5.000000000000001, "pose"={"Translation2d"={"x"=0.11563026000817181, "y"=0.15653335595178003}, "Rotation2d"={"Theta"=-0.022237140076929274}}, "curvature"=35.670320338983046}, {"t"=1.636809878720745, "velocity"=0.0, "acceleration"=-5.000000000000001, "pose"={"Translation2d"={"x"=0.11687890518731979, "y"=0.15652407853881273}, "Rotation2d"={"Theta"=-1.103625459485953e-14}}, "curvature"=-1.0970671007627583e-12}], 6 "Reverse Path?":bool)   [LabVIEW 2019]
uses:
  AutonBuilder/Typedef/Data Point.ctl
  <vilib>/Rock Robotics/WPI/ThirdParty/WPILib Extensions/Trajectory/Typedef/Trajectory State.ctl
  <vilib>/Rock Robotics/WPI/ThirdParty/WPILib Extensions/Geometry/Typedef/Pose2d.ctl
  <vilib>/Rock Robotics/WPI/ThirdParty/WPILib Extensions/Geometry/Typedef/Translation2d.ctl
  <vilib>/Rock Robotics/WPI/ThirdParty/WPILib Extensions/Geometry/Typedef/Rotation2d.ctl
panel:
  out "Total Time (s)":dbl=1.636809878720745
  out "Graph":cluster{dbl[], dbl[]}[](graph)=[{[2.848, 3.548, 3.548, 2.848, 2.848], [7.62, 7.62, 7.0200000000000005, 7.0200000000000005, 7.62]}, {[3.048, 6.688056195965419, 3.7631959654178675, 4.191678674351586, 4.601531700288184, 5.141792507204611], [7.32, 5.843945205479453, 6.124904109589042, 7.417315068493152, 6.162365296803654, 7.417315068493152]}, {array[201 elements], array[201 elements]}, {array[201 elements], array[201 elements]}, {array[201 elements], array[201 elements]}]
  in  "Data Points":T5[](array[typedef])=[{"X"=3.048, "Y"=7.32, "Theta"=0.0, "Speed %"=0.0, "Disabled?"=FALSE}, {"X"=6.688056195965419, "Y"=5.843945205479453, "Theta"=0.0, "Speed %"=0.0, "Disabled?"=TRUE}, {"X"=3.7631959654178675, "Y"=6.124904109589042, "Theta"=0.0, "Speed %"=0.0, "Disabled?"=FALSE}, {"X"=4.191678674351586, "Y"=7.417315068493152, "Theta"=0.0, "Speed %"=0.0, "Disabled?"=FALSE}, {"X"=4.601531700288184, "Y"=6.162365296803654, "Theta"=0.0, "Speed %"=0.0, "Disabled?"=FALSE}, {"X"=5.141792507204611, "Y"=7.417315068493152, "Theta"=0.0, "Speed %"=0.0, "Disabled?"=TRUE}]
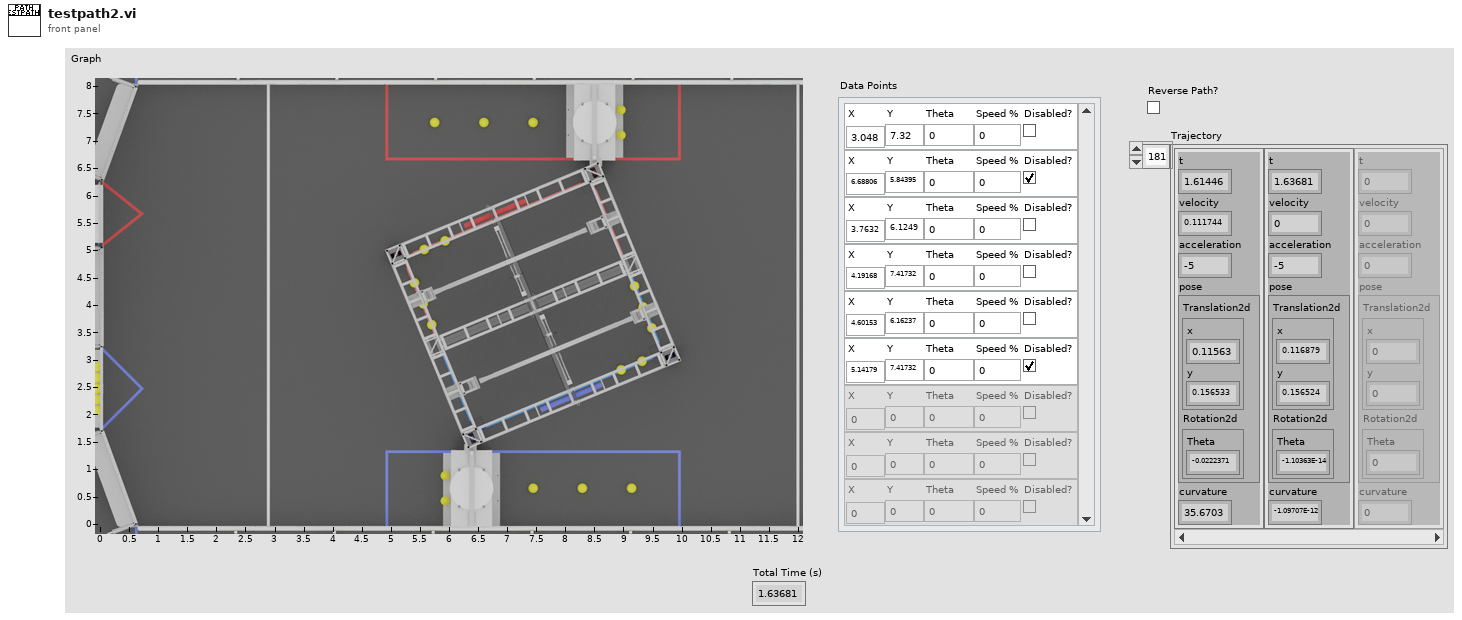
[diagram p1: front panel]
types:
  T1 = typedef "Trajectory State.ctl" = cluster{"t":dbl, "velocity":dbl, "acceleration":dbl, "pose":T2, "curvature":dbl}
  T2 = typedef "Pose2d.ctl" = cluster{"Translation2d":T3, "Rotation2d":T4}
  T3 = typedef "Translation2d.ctl" = cluster{"x":dbl, "y":dbl}
  T4 = typedef "Rotation2d.ctl" = cluster{"Theta":dbl}
  T5 = typedef "Data Point.ctl" = cluster{"X":dbl, "Y":dbl, "Theta":dbl, "Speed %":dbl, "Disabled?":bool}
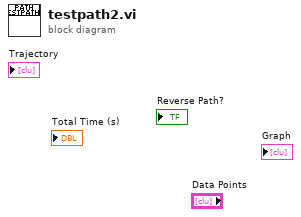
[diagram p0: block diagram]
diagram:
